vi "Build Unregister Message.vi"(0 "Target CSM":string, 5 "Source CSM (* as Default)":string="*", 7 "Status":string, 9 "API (* as Default)":string="*") -> (6 "CSM Message String":string)   [LabVIEW 2017, in "Communicable State Machine.lvlib"]
doc: "Concatenates unregister state operation message strings. The message format is as follows:\n\n //[source-state]@[source-module] >> [response-message]@[response-module] -><unregister>\n status @ Source >> API @ Target -><unregister>\n\n Example: Cancel the binding of the \"Download Finished\" message of the Downloader module to the \"Start Play\" API of the Player module.\n // Cancel binding of the \"Download Finished\" message of the Downloader module to the \"Start Play\" API of the Player module\n DownloadFinished@Downloader >> StartPlay@Player -><unregister>\n // When executing the message within the Player module, \"Player\" can be omitted\n DownloadFinished@Downloader >> StartPlay -><unregister>\n\n- In Worker Mode, the module's internal registration rules will only be automatically unregistered after all nodes have exited.\n- In Chain of Responsibility Mode, the module's internal registration rules will be automatically unregistered as the node exits.\n\n\n> [!NOTE] <b>Message Building API</b>\n>\n> This type of API is only used to concatenate message strings and does not send messages directly. The strings need to be merged into the CSM state queue, and the messages will be sent and the operation executed within the Parse State Queue++ VI. If you are familiar with CSM rules, you do not need to use this type of API. You can type the corresponding message string or operation string directly into the string.\n\n\n> [!NOTE] <b>CSM Registration</b>\n>\n> Registration associates a broadcast with a bound interface (API). When the broadcast is triggered, the bound interface (API) is called. Registrations can also be cancelled. In CSM, there are two types of broadcasts:\n>\n> - <b>Broadcast</b>: Broadcast explicitly called by the module sending the broadcast message. Arguments need to be explicitly provided.\n> - <b>State</b>: Any state of a CSM module can also be registered to. The argument received by the triggered API is the Response of the CSM state.\n>\n> // Register\n> [CSM Broadcast]@[SourceModule] >> [Bound API]@[TargetModule] -><register> // [Comments]\n> // Unregister\n> [CSM Broadcast]@[SourceModule] >> [Bound API]@[TargetModule] -><unregister> // [Comments]\n>\n> - <b>CSM Broadcast</b>: Defined by the source module. Refer to \"CSM Broadcast Format Parsing\" for details.\n> - <b>Source Module</b>: The broadcasting module. If registering to broadcasts from any module, the source module can be represented by `*`.\n> - <b>Bound API</b>: Defined by the target module. It is the external interface of the target module.\n> - <b>Target Module</b>: The module where the bound API resides. When indicating registration to the current module within a CSM module, it can be ignored. The preceding `@` separator is also omitted.\n> - `<register>` / `<unregister>`: Definition of the Register/Unregister operation type.\n> - <b>Comments</b>: Comment information, which will not be parsed.\n\n\n> [!NOTE] <b>CSM Registration Location</b>\n>\n> There are two types of registration rules added by CSM registrations: Internal Addition and External Addition.\n> - <b>External Addition</b>: Rules added externally are global rules. They will not be automatically deleted when the CSM module exits and must be manually unregistered.\n> - Rules added using the `-<register>` statement are considered externally added if the module name where the API resides is specified.\n> - All rules added using the API CSM - Register Broadcast VI are considered externally added.\n> - <b>Internal Addition</b>: Rules added internally within a CSM module will be automatically deleted when the CSM module exits, so there is no need to manually unregister.\n> - Rules are considered internally added only when added using the `-<register>` statement and the API does not specify a module name.\n>\n> // Example:\n> status@sourceModule >> API@TargetModule -><register> // Externally added\n> status@sourceModule >> API -><register> // Internally added\n\n\n-- <b>Controls</b> --\n- <b>Target CSM</b>: Name of the CSM module registering to the status.\n- <b>Source CSM (* as Default)</b>: Name of the CSM module publishing the status.\n- <b>Status</b>: Registered status.\n- <b>API (If \"\", Same As \"Status\")</b>: Name of the API in the registering module that responds to the status to be unregistered.\n\n-- <b>Indicators</b> --\n- <b>CSM Message String</b>: Concatenated CSM message string."
uses:
  Communicable State Machine.lvlib
  _Shared/CSM Shared.lvlib
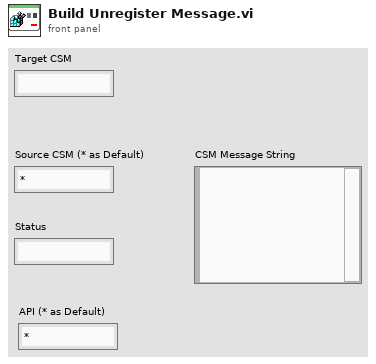
[diagram p1: front panel]
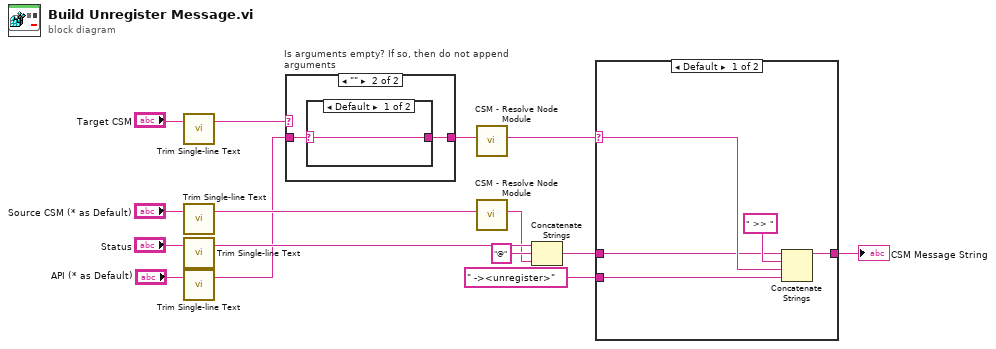
[diagram p0: block diagram]
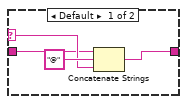
[diagram p2: hidden frame]
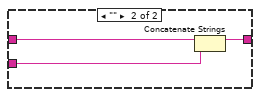
[diagram p4: hidden frame]
diagram:
  n1 = call "Trim Single-line Text.vi"("single-line text"="Target CSM") -> ("trimed text"=w5:string)  [unwired: 2 in]
  n2 = call "Trim Single-line Text.vi"("single-line text"="Source CSM (* as Default)") -> ("trimed text"=w9:string)  [unwired: 2 in]
  n3 = call "Trim Single-line Text.vi"("single-line text"="Status") -> ("trimed text"=w11:string)  [unwired: 2 in]
  n4 = call "Trim Single-line Text.vi"("single-line text"="API (* as Default)") -> ("trimed text"=w3:string)  [unwired: 2 in]
  n5 = case "Is arguments empty? If so, then do not append arguments" shown="\"\"" w5 {
    selector: w5 -> [w17 _]
    tunnel: [w18 w20] -> w4
    tunnel: w3 -> [w16 w21]
    frame Default {
      n6 = Concatenate Strings(w16, "@" ("string"), w17) -> (w18:string)
    }
    frame "" {
      n7 = case shown="Default" w21 {
        selector: w21 -> [w22 _]
        tunnel: [w22 _] -> w20
        frame Default {
        }
        frame "*" {
        }
      }
    }
  }
  n8 = call "CSM - Resolve Node Module.vi"("Node Name"=w4) -> ("CSM Module Name"=w1:string)  [unwired: 10 in]
  n9 = call "CSM - Resolve Node Module.vi"("Node Name"=w9) -> ("CSM Module Name"=w2:string)  [unwired: 10 in]
  n10 = Concatenate Strings(w11, "@" ("string"), w2) -> (w8:string)
  n11 = case shown="Default" w1 {
    selector: w1 -> [w26 _]
    tunnel: [w27 w30] -> w15
    tunnel: w8 -> [w24 w29]
    tunnel: " -><unregister>" ("string") -> [w23 w28]
    frame Default {
      n12 = Concatenate Strings(w24, " >> " ("string"), w26, w23) -> (w27:string)
    }
    frame "" {
      n13 = Concatenate Strings(w29, w28) -> (w30:string)
    }
  }
  "CSM Message String" <- w15
